vi "Get Current Mouse Lat Lon.vi"(8 "error in (no error)":errorcluster, 11 "This VI":refnum<vi>) -> (0 "Error Out":errorcluster, 1 "Lon":dbl, 2 "Lat":dbl, 3 "Point Ref":refnum<k24>)   [LabVIEW 2014]
uses:
  C:/Robotic Systems/Products/Surveyor/Software/Ground Station/Data/Mapping DLL/GMap.NET.Core.dll
  Data/Mapping DLL/GMap.NET.Core.dll
  <vilib>/Utility/miscctls.llb/LVPositionTypeDef.ctl
  USER32.DLL
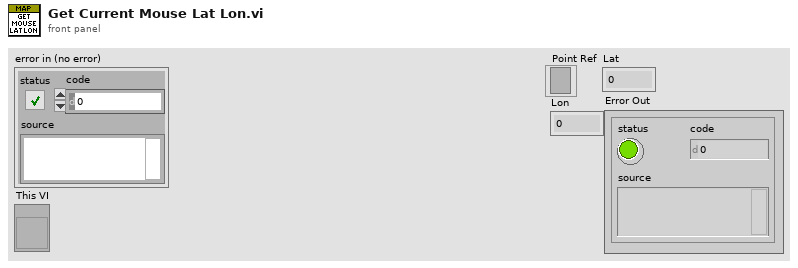
[diagram p1: front panel]
types:
  T1 = typedef "LVPositionTypeDef.ctl" = cluster{"Left":i32, "Top":i32}
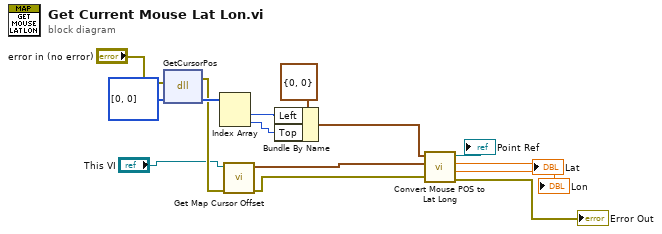
[diagram p0: block diagram]
diagram:
  n1 = dll-call lib="USER32.DLL" fn="GetCursorPos"(error in="error in (no error)", "Position"=i32[] [0, 0]) -> (error out=w8:errorcluster, "Position"=w15:i32[])  [unwired: 3 in, 1 out]
  n2 = Index Array(array=w15) -> (element #1=w12:i32, element #2=w11:i32)  [unwired: 2 in]
  n3 = call "Get Map Cursor Offset.vi"("error in (no error)"=w8, "This VI"="This VI") -> ("error out"=w7:errorcluster, "Gmap Offset"=w9:T1)  [unwired: 8 in]
  n4 = Bundle By Name(cluster=T1 {"Left"=0, "Top"=0} ("Mouse Position"), "Left"=w12, "Top"=w11) -> (w10:T1)
  n5 = call "Convert Mouse POS to Lat Long.vi"("Error In"=w7, "GMap Position"=w9, "Mouse Position"=w10) -> ("Error Out"=→"Error Out":errorcluster, "Lng"=→"Lon":dbl, "Lat"=→"Lat":dbl, "Point Ref"=→"Point Ref":refnum<k24>)  [unwired: 5 in]
